vi "Discovery2.vi"() -> ()   [LabVIEW 2015]
uses:
  DigilentWF/DigilentWF.lvlib
panel:
  in  "Channel 2":string caption="Channel"
  in  "Enable Tracking":bool
  out "Error Out 2":errorcluster
  in  "Enable Outputs":bool
  out "Error Out":errorcluster
  in  "Current Limit":dbl(knob)=0.1026571496540006 caption="Current Limit (no change)" scale=0.0..0.7
  in  "Voltage Level":dbl(knob) caption="Voltage Level (no change)" scale=0.0..5.0
  in  "Channel":string
  in  "Stop Button":bool
  in  "Device Name":string="Discovery2"
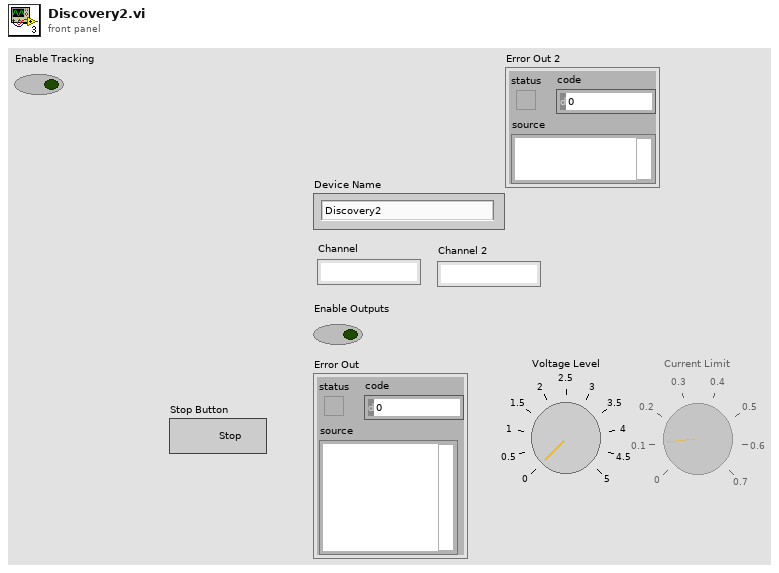
[diagram p1: front panel]
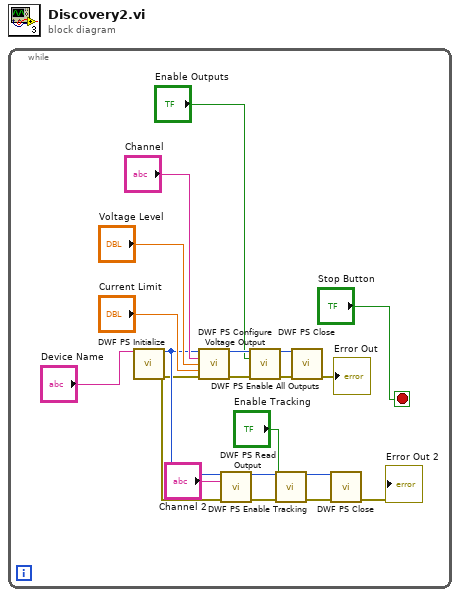
[diagram p0: block diagram]
diagram:
  n1 = while {
    stop <- "Stop Button" stop-if-true
    n2 = call <vilib>:"DWF PS Initialize.vi"("Device Name"="Device Name") -> ("Instrument Handle Out"=w10:u32, "Error Out"=w9:errorcluster)  [unwired: 13 in]
    n3 = call <vilib>:"DWF PS Configure Voltage Output.vi"("Instrument Handle In"=w10, "Channel"="Channel", "Voltage Level"="Voltage Level", "Current Limit"="Current Limit", "Error In"=w9) -> ("Instrument Handle Out"=w19:u32, "Error Out"=w17:errorcluster)  [unwired: 9 in]
    n4 = call <vilib>:"DWF PS Read Output.vi"("Instrument Handle In"=w10, "Channel"="Channel 2", "Error In"=w9) -> ("Instrument Handle Out"=w11:u32, "Error Out"=w8:errorcluster)  [unwired: 8 in, 3 out]
    n5 = call <vilib>:"DWF PS Enable All Outputs.vi"("Instrument Handle In"=w19, "Enable Outputs"="Enable Outputs", "Error In"=w17) -> ("Instrument Handle Out"=w2:u32, "Error Out"=w1:errorcluster)  [unwired: 11 in]
    n6 = call <vilib>:"DWF PS Enable Tracking.vi"("Instrument Handle In"=w11, "Enable Tracking"="Enable Tracking", "Error In"=w8) -> ("Instrument Handle Out"=w6:u32, "Error Out"=w7:errorcluster)  [unwired: 11 in]
    n7 = call <vilib>:"DWF PS Close.vi"("Instrument Handle In"=w2, "Error In"=w1) -> ("Error Out"=→"Error Out":errorcluster)  [unwired: 13 in]
    n8 = call <vilib>:"DWF PS Close.vi"("Instrument Handle In"=w6, "Error In"=w7) -> ("Error Out"=→"Error Out 2":errorcluster)  [unwired: 13 in]
  }
